vi "基恩士PLC测试软件.vi"() -> ()   [LabVIEW 2017]
panel:
  out "数据输出":string
  in  "服务器关闭":string="服务器VI关闭了连接。"
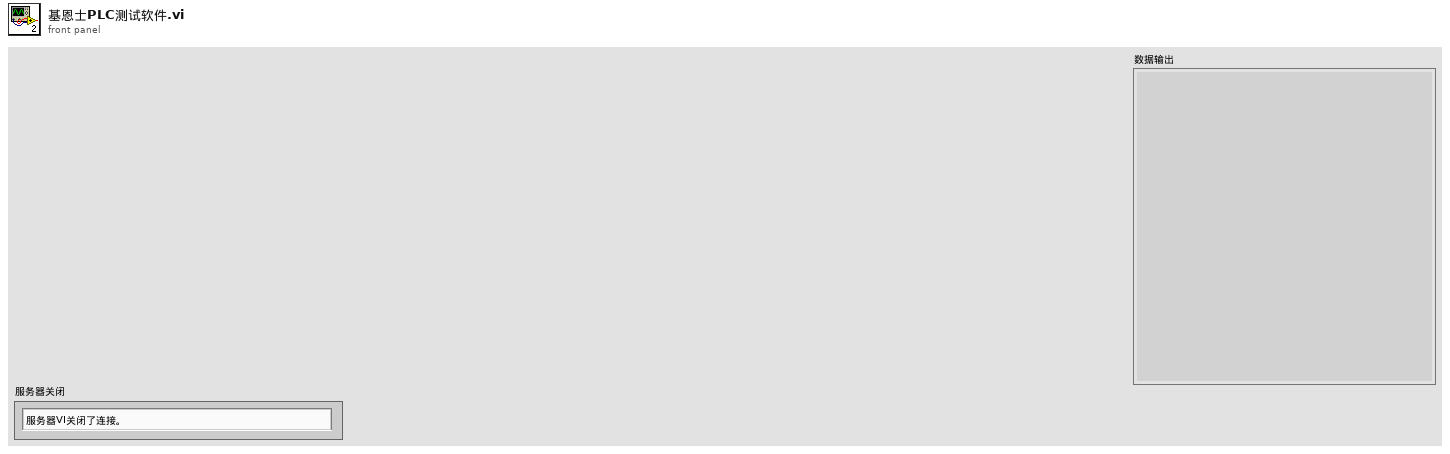
[diagram p1: front panel]
types:
  T1 = enum16{"Standard", "Buffered", "CRLF", "Immediate"}
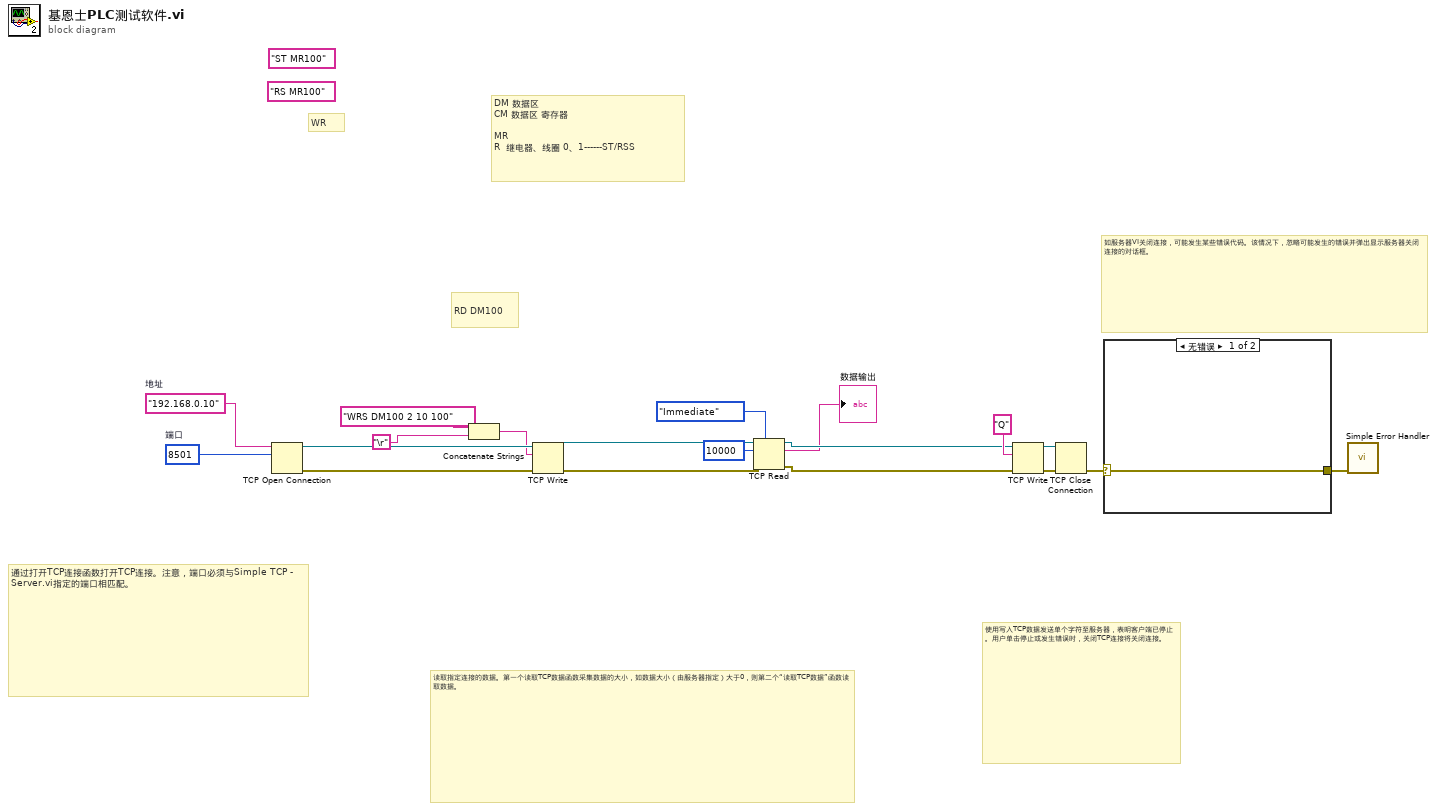
[diagram p0: block diagram]
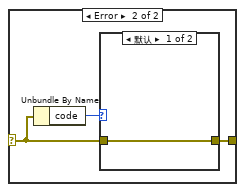
[diagram p2: hidden frame]
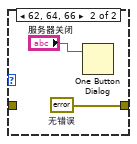
[diagram p3: hidden frame]
diagram:
  (unwired) "RS MR100"
  (unwired) "ST MR100"
  w11 = u16 8501  # 端口
  w12 = "192.168.0.10"  # 地址
  # "DM 数据区\nCM 数据区 寄存器\n\nMR\nR  继电器、线圈 0、1------ST/RSS"
  # "WR"
  # "如服务器VI关闭连接，可能发生某些错误代码。该情况下，忽略可能发生的错误并弹出显示服务器关闭连接的对话框。"
  # "使用写入TCP数据发送单个字符至服务器，表明客户端已停止。用户单击停止或发生错误时，关闭TCP连接将关闭连接。"
  # "读取指定连接的数据。第一个读取TCP数据函数采集数据的大小，如数据大小（由服务器指定）大于0，则第二个“读取TCP数据”函数读取数据。"
  # "通过打开TCP连接函数打开TCP连接。注意，端口必须与Simple TCP - Server.vi指定的端口相匹配。"
  # "RD DM100"
  n1 = TCP Open Connection(address=w12, remote port or service name=w11) -> (connection ID=w19:refnum<k5>, error out=w18:errorcluster)  [unwired: 3 in]
  n2 = Concatenate Strings("WRS DM100 2 10 100", "\r") -> (w6:string)
  n3 = TCP Write(connection ID=w19, data in=w6, error in (no error)=w18) -> (connection ID out=w5:refnum<k5>, error out=w4:errorcluster)  [unwired: 1 in, 1 out]
  n4 = TCP Read(connection ID=w5, bytes to read=10000 ("读取的字节"), error in (no error)=w4, 7:T1."Immediate" ("模式（标准）")) -> (connection ID out=w9:refnum<k5>, data out=→"数据输出":string, error out=w10:errorcluster)  [unwired: 1 in]
  n5 = TCP Write(connection ID=w9, data in="Q", error in (no error)=w10) -> (connection ID out=w17:refnum<k5>, error out=w16:errorcluster)  [unwired: 2 out]
  n6 = TCP Close Connection(connection ID=w17, error in (no error)=w16) -> (error out=w14:errorcluster)  [unwired: 1 in, 1 out]
  n7 = case shown="无错误" w14 {
    selector: w14 -> [w20 w22]
    tunnel: [w20 w21] -> w13
    frame No Error {
    }
    frame Error {
      n8 = Unbundle By Name(w22) -> ("code"=w23:i32)
      n9 = case shown="默认" w23 {
        tunnel: w22 -> [w24 _]
        tunnel: [w24 w26] -> w21
        frame Default {
        }
        frame 62, 64, 66 {
          w26 = errorcluster {"status"=FALSE, "code"=0, "source"=""}  # 无错误
          n10 = One Button Dialog(message="服务器关闭") -> ()  [unwired: 1 in, 1 out]
        }
      }
    }
  }
  n11 = call <vilib>:"Simple Error Handler.vi"("error in (no error)"=w13) -> ()  [unwired: 4 in, 5 out]
